vi "Handling Return Dictionaries.vi"() -> ()   [LabVIEW 2020, in "OPI.lvclass"]
uses:
  OPI.lvclass
  Typedefs/Cmd Line Mode.ctl
  Get Return/Get Return - Pythonic.vi
  From Pythonic/From Pythonic - Dictionary.vi
  From Pythonic/From Pythonic - Float.vi
  From Pythonic/From Pythonic - Integer.vi
  From Pythonic/From Pythonic - Boolean.vi
panel:
  out "Float":dbl
  out "Integer":i64
  out "Return Value":bool caption="Boolean"
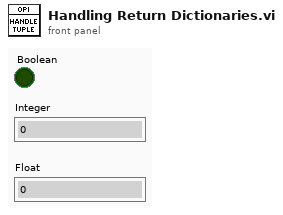
[diagram p1: front panel]
types:
  T1 = typedef "OPI.lvclass/Cmd Line Mode.ctl" = enum16{"Debug", "Hidden"}
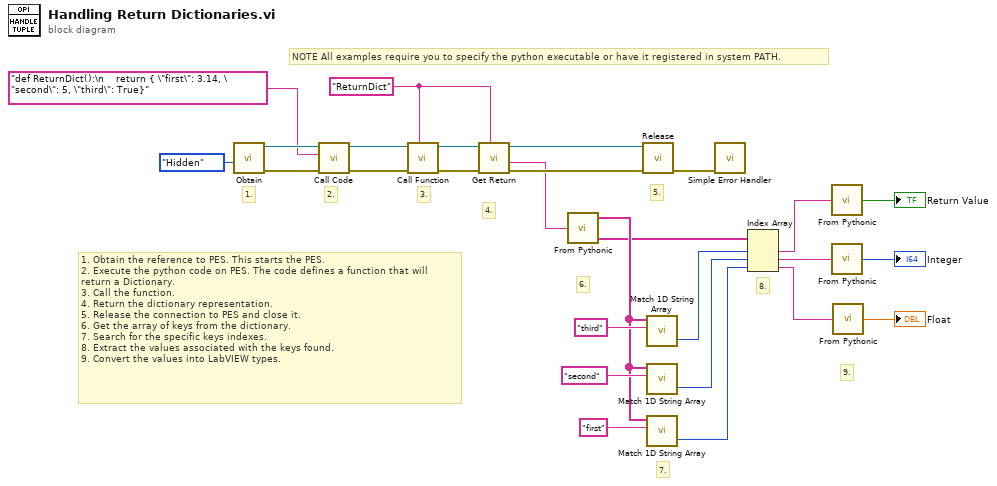
[diagram p0: block diagram]
diagram:
  w18 = "ReturnDict" ("Function")
  # "NOTE All examples require you to specify the python executable or have it registered in system PATH."
  # "9."
  # "8."
  # "1. Obtain the reference to PES. This starts the PES.\n2. Execute the python code on PES. The code defines a function that will\nreturn a Dictionary.\n3. Call the function.\n4. Return the dictionary representation.\n5. Release the connection to PES and close it.\n6. Get the array of keys from the dictionary.\n7. Search for the specific keys indexes.\n8. Extract the values associated with the keys found.\n9. Convert the values into LabVIEW types."
  # "7."
  # "6."
  # "5."
  # "4."
  # "3."
  # "2."
  # "1."
  n1 = call "Obtain.vi"("Cmd Line Mode (Hidden)"=Cmd_Line_Mode."Hidden") -> ("Error Out"=w26:errorcluster, "OPI Ref"=w27:refnum<data-value>)  [unwired: 9 in]
  n2 = call "Call Code.vi"("Error In"=w26, "Pythonic Code"="def ReturnDict():\n    return { \"first\": 3.14, \"second\": 5, \"third\": True}", "OPI Ref"=w27) -> ("Error Out"=w23:errorcluster, "OPI Ref"=w24:refnum<data-value>)  [unwired: 7 in]
  n3 = call "Call Function.vi"("Function Name"=w18, "Error In"=w23, "OPI Ref"=w24) -> ("Error Out"=w19:errorcluster, "OPI Ref"=w20:refnum<data-value>)  [unwired: 7 in]
  n4 = call-poly "Get Return.vi"("Function Name"=w18, "Error In"=w19, "OPI Ref"=w20) -> ("Error Out"=w14:errorcluster, "Pythonic Return Value"=w3:string, "OPI Ref"=w22:refnum<data-value>)  [unwired: 6 in]
  n5 = call-poly "From Pythonic.vi"("Pythonic Value"=w3) -> ("Values"=w1:string[], "Keys"=w2:string[])  [unwired: 3 in]
  n6 = call "Release.vi"("Error In"=w14, "OPI Ref"=w22) -> ("Error Out"=w13:errorcluster)  [unwired: 9 in]
  n7 = call <vilib>:"Match 1D String Array.vi"("Pattern"="third", "Strings"=w2) -> ("index of element"=w12:i32)  [unwired: 2 in, 1 out]
  n8 = call <vilib>:"Match 1D String Array.vi"("Pattern"="second", "Strings"=w2) -> ("index of element"=w11:i32)  [unwired: 2 in, 1 out]
  n9 = call <vilib>:"Match 1D String Array.vi"("Pattern"="first", "Strings"=w2) -> ("index of element"=w10:i32)  [unwired: 2 in, 1 out]
  n10 = call <vilib>:"Simple Error Handler.vi"("error in (no error)"=w13) -> ()  [unwired: 4 in, 5 out]
  n11 = Index Array(array=w1, index #1=w12, index #2=w11, index #3=w10) -> (element #1=w4:string, element #2=w6:string, element #3=w5:string)
  n12 = call-poly "From Pythonic.vi"("Pythonic Value"=w4) -> ("Boolean"=→"Return Value":bool)  [unwired: 4 in]
  n13 = call-poly "From Pythonic.vi"("Pythonic Value"=w6) -> ("Integer"=→"Integer":i64)  [unwired: 4 in]
  n14 = call-poly "From Pythonic.vi"("Pythonic Value"=w5) -> ("Float"=→"Float":dbl)  [unwired: 4 in]
